vi "Main.vi"(11 "Module Admin":refnum<class "Delacor_lib_QMH_Module Admin.lvclass">) -> ()   [LabVIEW 2022 SP3, in "StateMachine.lvlib"]
doc: "This template is based off of the default DQMH. It implements the HSE Flavor of DQMH (see https://dokuwiki.hampel-soft.com/code/dqmh/hse-flavour) and adds a state machine to the module.\n\nThe state machine is based off of SSDC's (http://www.ssdc.co.uk/) state machine template. \n____\nHAMPEL SOFTWARE ENGINEERING v2.6.0 (2023-12-19 10:54)"
uses:
  StateMachine.lvlib
  <vilib>/Delacor/Delacor QMH/Libraries/Module Admin_class/Delacor_lib_QMH_Module Admin.lvclass
  HSE-SM/SM_States.ctl
  HSE-SM/SM_Transitions.ctl
  Module Data--cluster.ctl
  Libraries/hse-libraries/Source/hse-dqmh/Controls/Module Display Scenarios.ctl
  <vilib>/Delacor/Delacor QMH/Libraries/Module Admin_class/Delacor_lib_QMH_Module Admin.lvclass/Delacor_lib_QMH_Module Admin.ctl
  Configure Argument--cluster.ctl
  <vilib>/Delacor/Delacor QMH/Libraries/Message Queue_class/Delacor_lib_QMH_Message Queue.lvclass/Delacor_lib_QMH_Message Queue.ctl
  Prepare Argument--cluster.ctl
  Request UI Display Argument--cluster.ctl
  Request UI Display (Reply Payload)--cluster.ctl
  DEMO Inject Transition Argument--cluster.ctl
  Stop Argument--cluster.ctl
  <vilib>/Utility/miscctls.llb/LVPointTypeDef.ctl
  <vilib>/Delacor/Delacor QMH/Libraries/Message Queue_class/Delacor_lib_QMH_Enqueue Message (Single).vi
  <vilib>/Delacor/Delacor QMH/Libraries/Module Admin_class/Delacor_lib_QMH_Get External Launch.vi
  <vilib>/Utility/error.llb/Error Cluster From Error Code.vi
  <vilib>/ErrorRing/Error Ring.xnode
  <vilib>/Delacor/Delacor QMH/Libraries/Message Queue_class/Delacor_lib_QMH_Message Queue.lvclass
  Libraries/hse-libraries/Source/hse-configuration/config-ini/config-ini.lvclass
  <vilib>/Hampel Software Engineering/HSE Logger/hse-logger.lvlib
  Libraries/hse-libraries/Source/hse-dqmh/hse-dqmh.lvlib
  HSE-SM/HSE-State-Machine.lvlib
  Framework/UI Manager/UI Manager.lvlib
panel:
  in  "Nested Logic: Skip Polling?":bool caption="Skip Polling?"
  in  "Request Transition":T1
  in  "Polling Loop Signal":bool
  out "Current State":T2
  out "SM Exception":errorcluster
  out "error out":errorcluster
  # "The \"HSE State Machine Module\" serves as an example of how to use our HSE State Machine reference\narchitecture.\n\nThe module features a helper loop which hosts the state machine. Each state has a number of transitions\nit will process: Transitions can either lead to other states, be ignored, or even throw an error.\n\nBy default, states wait for transitions. Alternatively, there's the concept of \"polling states\".  Transitions \nare meant to be results of either the change of state of the system or triggered by user actions.\n\nUse the \"Request Transition\" enumerator to trigger transitions manually and observe how the state \nmachine reacts by watching the \"Current State\" indicator. Use the Skip Polling? and Polling Loop Signal \ncontrols accordingly to further manipulate the state machine."
  # "ENLARGE WINDOW TO SEE STATE CHART"
  # "See block diagram for details on this."
  # "Set this control to request a transition to the \nstate machine and observe its reaction with \nthe Current State indicator. \"Exit\" will close \nthe whole application."
  # "Set this control to \"true\" to satisfy the polling\ncondition and make the state machine leave\nthe polling state \"Polling for Signal Change\"."
  # "notice that the state machine doesn't allow the module to stop in every state and \nthat we didn't draw exception transitions."
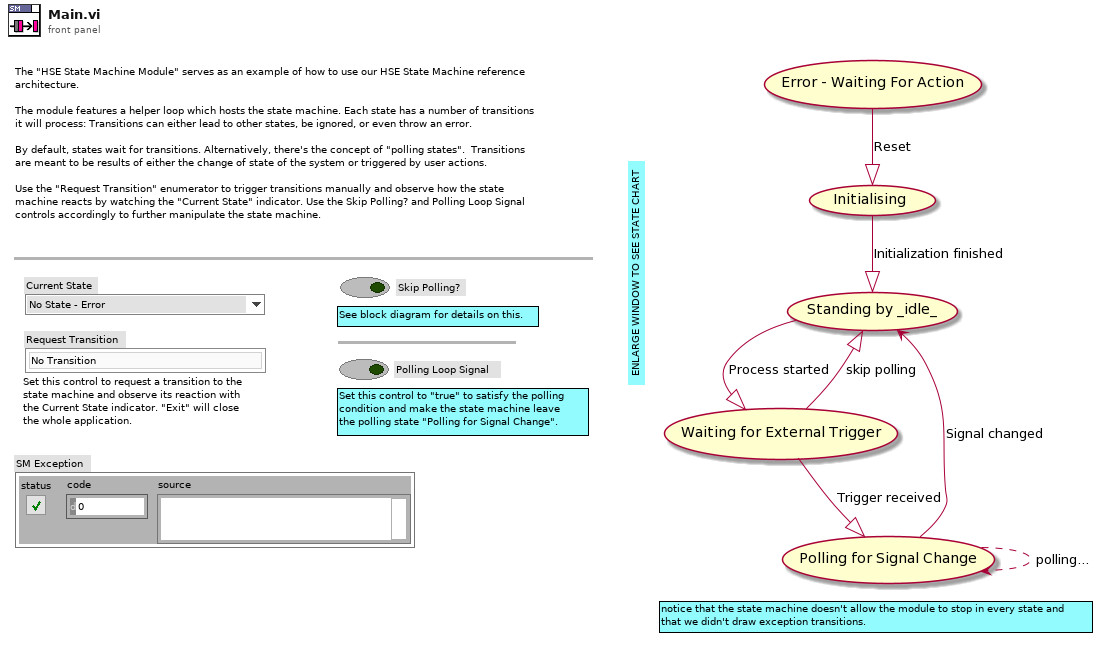
[diagram p1: front panel]
types:
  T1 = typedef "StateMachine.lvlib/HSE-State-Machine.lvlib/SM_Transitions.ctl" = enum16{"No Transition", "Exception", "Reset", "Initialization finished", "Process started", "Trigger detected", "Exit"}
  T2 = typedef "StateMachine.lvlib/HSE-State-Machine.lvlib/SM_States.ctl" = enum16{"No State - Error", "Error - Waiting For Action", "Initialising", "Standing by (idle)", "Waiting for External Trigger", "Polling for Signal Change", "Exiting"}
  T3 = typedef "StateMachine.lvlib/Request Events--cluster.ctl" = cluster{"Stop Module":refnum<user-event>, "Show Panel":refnum<user-event>, "Hide Panel":refnum<user-event>, "Get Module Execution Status":refnum<user-event>, "Show Diagram":refnum<user-event>, "Configure":refnum<user-event>, "Prepare":refnum<user-event>, "Request UI Display":refnum<user-event>, "DEMO Inject Transition":refnum<user-event>, "Exit EHL":refnum<user-event>}
  T4 = typedef "StateMachine.lvlib/Module Data--cluster.ctl" = cluster{"Scenario":T5}
  T5 = typedef "hse-dqmh.lvlib/Module Display Scenarios.ctl" = enum16{"Stand-Alone", "Managed"}
  T6 = typedef "StateMachine.lvlib/Stop Argument--cluster.ctl" = cluster{"Origin":string, "Exit via Stop Module Req?":bool, "Wait for Module to stop?":bool}
  T7 = enum32{"invalid lock state", "Not Locked", "Locked (No Password)", "Password-protected"}
  T8 = typedef "StateMachine.lvlib/Configure Argument--cluster.ctl" = cluster{"Boolean":bool}
  T9 = typedef "StateMachine.lvlib/Prepare Argument--cluster.ctl" = cluster{"Boolean":bool}
  T10 = typedef "StateMachine.lvlib/Request UI Display Argument--cluster.ctl" = cluster{"Scenario":T5, "Wait Notifier":refnum<notifier>, "wait for reply":bool}
  T11 = typedef "StateMachine.lvlib/DEMO Inject Transition Argument--cluster.ctl" = cluster{"Transition":T1, "Data":variant}
  T12 = typedef "LVPointTypeDef.ctl" = cluster{"Horizontal":i16, "Vertical":i16}
  T13 = enum32{"Invalid", "Standard", "Closed", "Hidden", "Minimized", "Maximized"}
  T14 = typedef "StateMachine.lvlib/Request UI Display (Reply Payload)--cluster.ctl" = cluster{"Accept?":bool, "error":errorcluster}
  T15 = typedef "StateMachine.lvlib/HSE-State-Machine.lvlib/SM Polling Actions--enum.ctl" = enum16{"Check transitions...", "Leave this state!"}
  T16 = typedef "hse-dqmh.lvlib/System Message Source.ctl" = enum16{"module", "application", "network"}
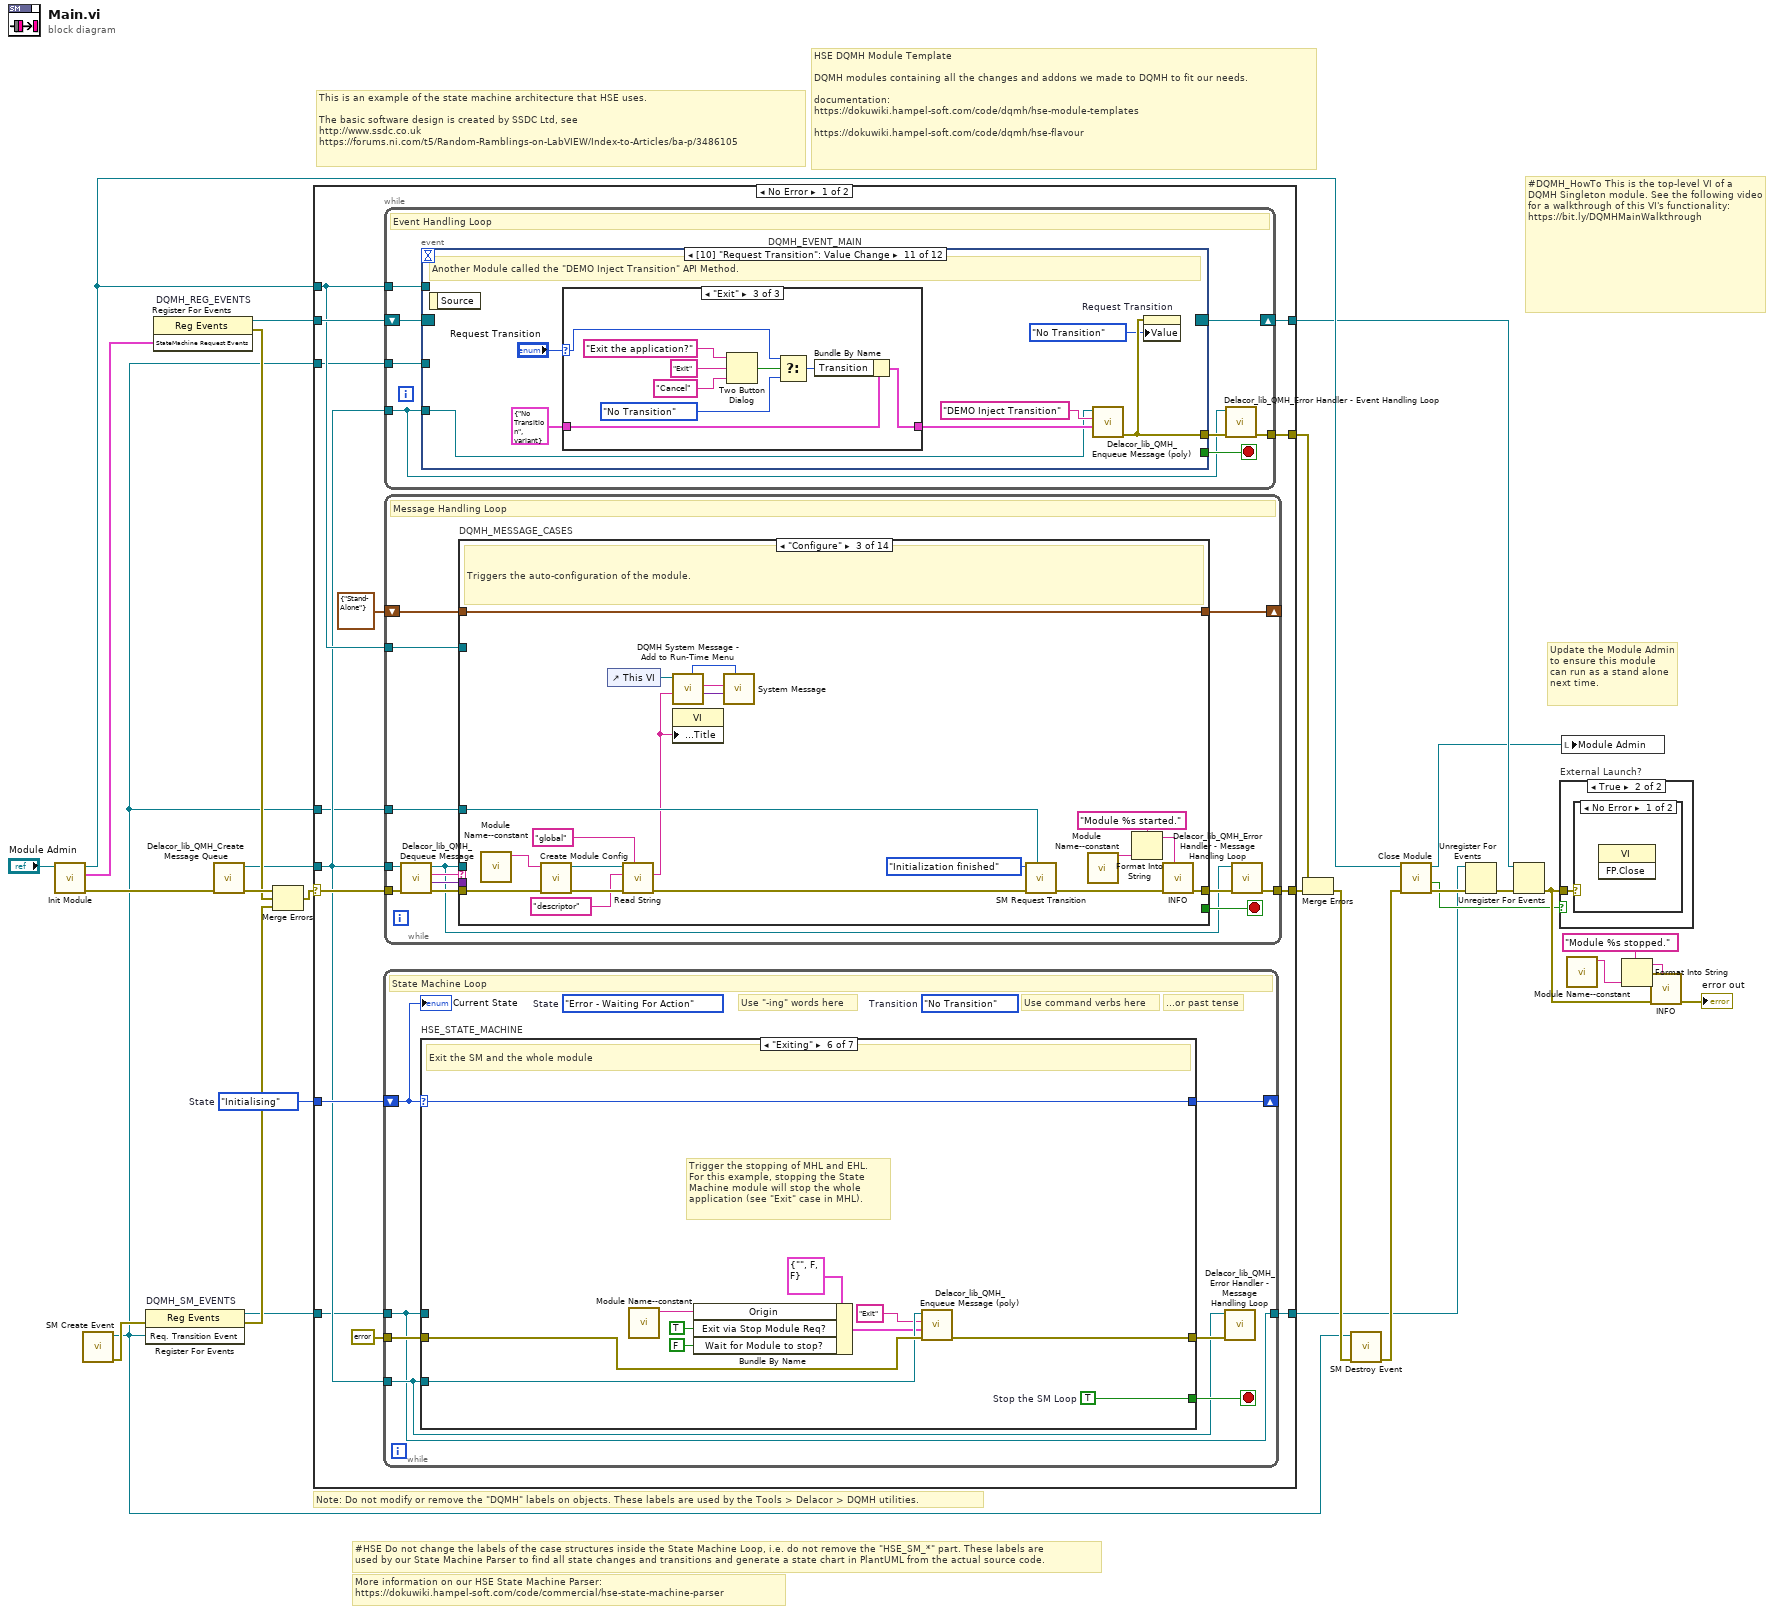
[diagram p0: block diagram]
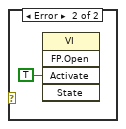
[diagram p3: hidden frame]
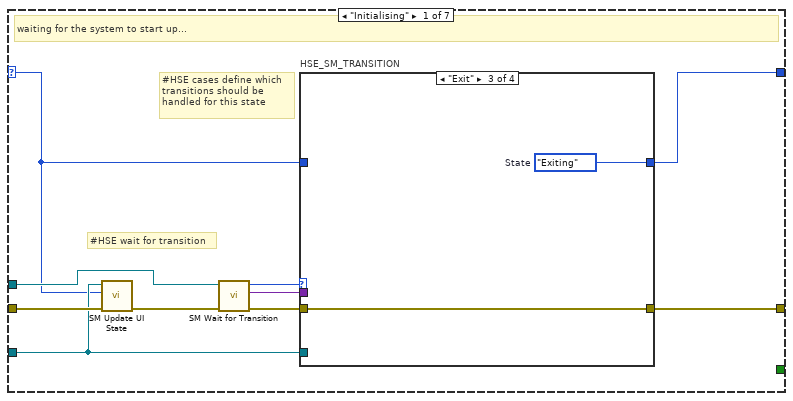
[diagram p4: hidden frame]
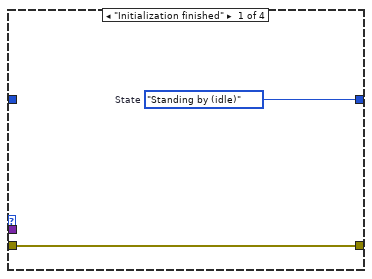
[diagram p5: hidden frame]
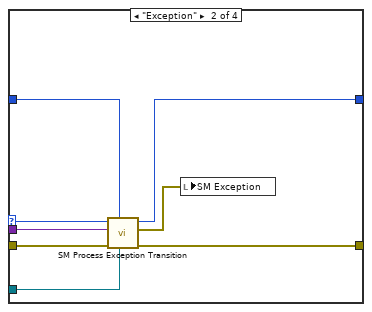
[diagram p6: hidden frame]
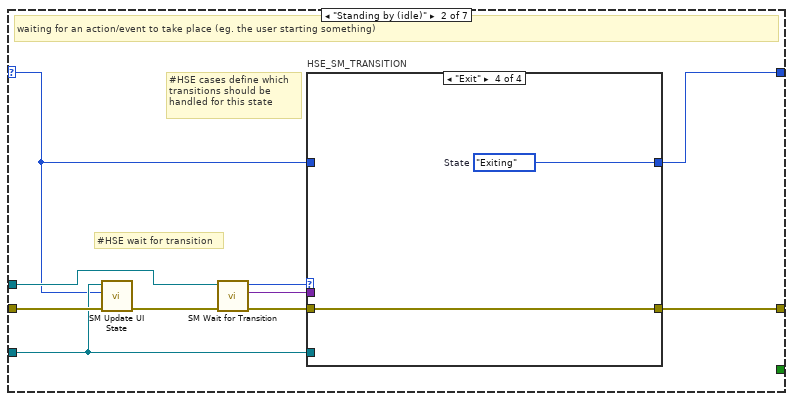
[diagram p8: hidden frame]
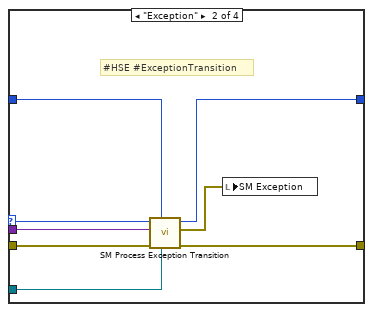
[diagram p10: hidden frame]
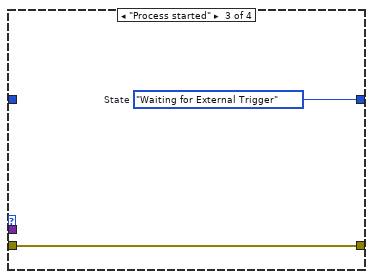
[diagram p11: hidden frame]
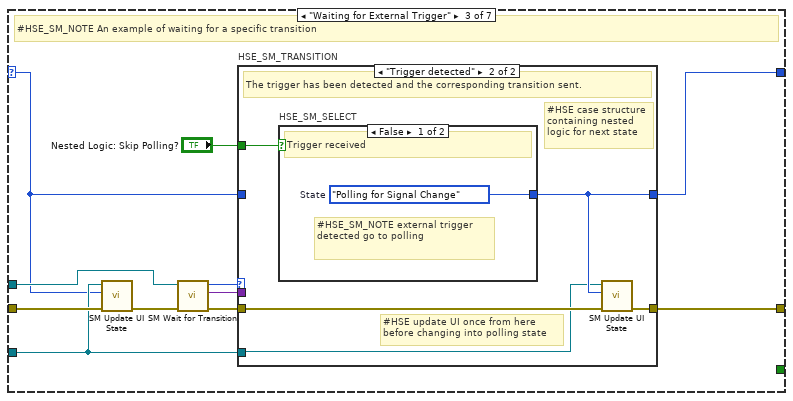
[diagram p12: hidden frame]
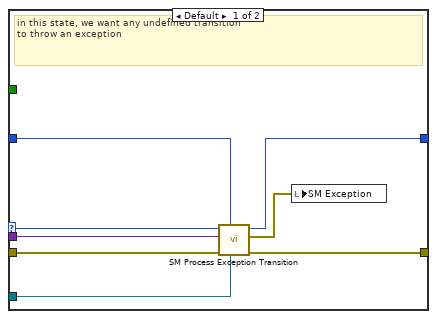
[diagram p13: hidden frame]
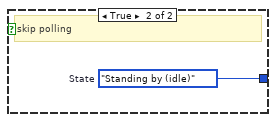
[diagram p14: hidden frame]
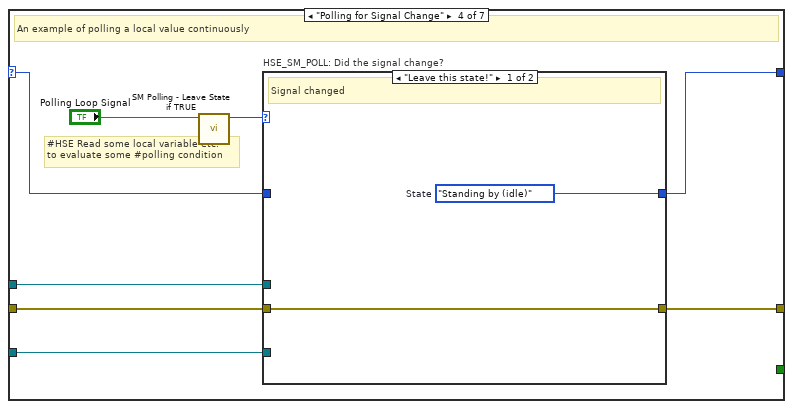
[diagram p15: hidden frame]
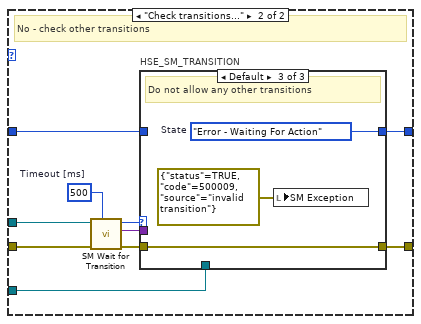
[diagram p16: hidden frame]
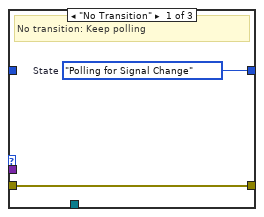
[diagram p17: hidden frame]
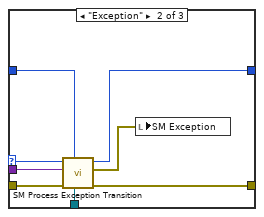
[diagram p18: hidden frame]
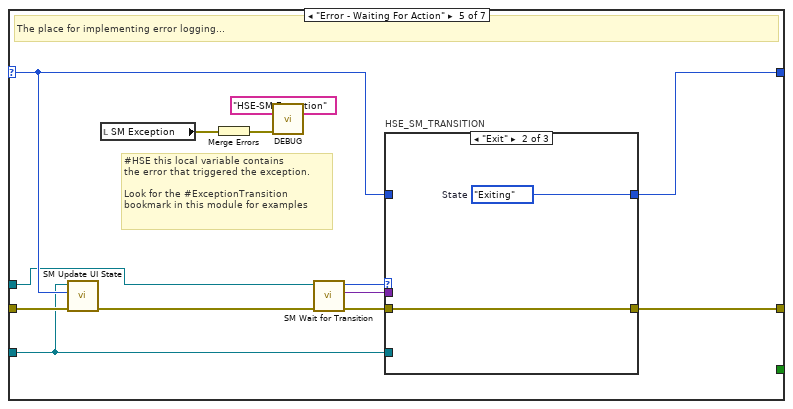
[diagram p19: hidden frame]
diagram:
  w12 = SM_States."Initialising"  # State
  # "More information on our HSE State Machine Parser: \nhttps://dokuwiki.hampel-soft.com/code/commercial/hse-state-machine-parser"
  # "#HSE Do not change the labels of the case structures inside the State Machine Loop, i.e. do not remove the \"HSE_SM_*\" part. These labels are\nused by our State Machine Parser to find all state changes and transitions and generate a state chart in PlantUML from the actual source code."
  # "HSE DQMH Module Template\n\nDQMH modules containing all the changes and addons we made to DQMH to fit our needs.\n\ndocumentation:\nhttps://dokuwiki.hampel-soft.com/code/dqmh/hse-module-templates\n\nhttps://dokuwiki.hampel-soft.com/code/dqmh/hse-flavour"
  # "This is an example of the state machine architecture that HSE uses. \n\nThe basic software design is created by SSDC Ltd, see \nhttp://www.ssdc.co.uk\nhttps://forums.ni.com/t5/Random-Ramblings-on-LabVIEW/Index-to-Articles/ba-p/3486105"
  # "#DQMH_HowTo This is the top-level VI of a DQMH Singleton module. See the following video for a walkthrough of this VI's functionality: https://bit.ly/DQMHMainWalkthrough"
  # "Note: Do not modify or remove the \"DQMH\" labels on objects. These labels are used by the Tools > Delacor > DQMH utilities."
  # "Update the Module Admin to ensure this module can run as a stand alone next time."
  n1 = call "Init Module.vi"("Singleton Module Admin in"="Module Admin") -> ("error out"=w27:errorcluster, "StateMachine Request Events"=w11:T3, "Singleton Module Admin out"=w23:refnum<class "Delacor_lib_QMH_Module Admin.lvclass">)  [unwired: 8 in]
  n2 = call "SM Create Event.vi"() -> ("error out"=w8:errorcluster, "Req. Transition Event"=w5:refnum<user-event>)  [unwired: 10 in]
  n3 = register-events "DQMH_SM_EVENTS"(error in=w8, w5) -> (reference out=w10:refnum<event-registration>, error out=w29:errorcluster)  [unwired: 1 in]
  n4 = register-events "DQMH_REG_EVENTS"(w11) -> (reference out=w21:refnum<event-registration>, error out=w24:errorcluster)  [unwired: 2 in]
  n5 = call <vilib>:"Delacor_lib_QMH_Create Message Queue.vi"("error in"=w27) -> ("error out"=w25:errorcluster, "Message Queue"=w20:refnum<class "Delacor_lib_QMH_Message Queue.lvclass">)  [unwired: 9 in]
  n6 = Merge Errors(w25, w24, w29) -> (w9:errorcluster)
  n7 = case shown="No Error" w9 {
    selector: w9 -> [w41 w468]
    tunnel: [w43 w467] -> w28
    tunnel: [w40 w473] -> w22
    tunnel: w21 -> [w38 w473]
    tunnel: w20 -> [w35 w466]
    tunnel: [w42 _] -> w26
    tunnel: w23 -> [w37 w469]
    tunnel: w12 -> [w36 _]
    tunnel: w10 -> [w34 w465]
    tunnel: w5 -> [w32 _]
    tunnel: w5 -> [w31 _]
    tunnel: [w30 w465] -> w1
    frame No Error {
      n8 = while {
        shift-right: [w49] -> _
        shift-left: w36 -> [w50]
        tunnel: w35 -> [w45]
        tunnel: w34 -> [w44]
        tunnel: errorcluster {"status"=FALSE, "code"=0, "source"=""} ("error out") -> [w46]
        tunnel: [w44] -> w30
        stop <- w48 stop-if-true
        (unwired) SM_States."Error - Waiting For Action"  # State
        (unwired) SM_Transitions."No Transition"  # Transition
        # "...or past tense"
        # "Use command verbs here"
        # "Use \"-ing\" words here"
        # "State Machine Loop"
        n9 = case "HSE_STATE_MACHINE" shown="\"Exiting\"" w50 {
          selector: w50 -> [w51 w75 w99 w125 w161 w184 _]
          tunnel: [w56 w80 w105 w131 w162 w184 w189] -> w49
          tunnel: [_ _ _ _ _ w187 w191] -> w48
          tunnel: w45 -> [w52 w76 w101 w129 w158 w186 _]
          tunnel: [w55 w79 w104 w130 w164 w185 errorcluster {"status"=TRUE, "code"=500001, "source"="SM called \"No State\"!"} ("error out")] -> w47
          tunnel: w44 -> [w53 w77 w102 w128 w160 _ _]
          tunnel: w46 -> [w60 w84 w109 w132 w170 w188 _]
          frame "Initialising" {
            # "#HSE cases define which\ntransitions should be \nhandled for this state"
            # "#HSE wait for transition"
            # "waiting for the system to start up..."
            n10 = call "SM Update UI State.vi"("error in (no error)"=w60, "State"=w51, "Message Queue In"=w52) -> ("error out"=w54:errorcluster)  [unwired: 7 in, 1 out]
            n11 = call "SM Wait for Transition.vi"("error in (no error)"=w54, "Event Registration Refnum"=w53) -> ("error out"=w58:errorcluster, "Data"=w57:variant, "Transition"=w59:T1)  [unwired: 7 in]
            n12 = case "HSE_SM_TRANSITION" shown="\"Exit\"" w59 {
              selector: w59 -> [_ w64 _ _]
              tunnel: w58 -> [w62 w70 w72 w73]
              tunnel: w57 -> [_ w69 _ _]
              tunnel: [w61 w68 w71 w74] -> w56
              tunnel: [w62 w67 w72 w73] -> w55
              tunnel: w52 -> [_ w65 _ _]
              tunnel: w51 -> [_ w63 _ w74]
              frame "Initialization finished" {
                w61 = SM_States."Standing by (idle)"  # State
              }
              frame "Exception" {
                n13 = call "SM Process Exception Transition.vi"("Message Queue In"=w65, "Exception State"=w63, "error in (no error)"=w70, "Data"=w69, "Exception Transition"=w64) -> ("error out"=w67:errorcluster, "Exception"=w66:errorcluster, "State"=w68:T2)  [unwired: 4 in]
                n14 = local write "SM Exception"(w66) -> ()
              }
              frame "Exit" {
                w71 = SM_States."Exiting"  # State
              }
              frame Default {
                # "we intentionally want to ignore silently every other transition\nin this case"
              }
            }
          }
          frame "Standing by (idle)" {
            # "#HSE cases define which\ntransitions should be \nhandled for this state"
            # "#HSE wait for transition"
            # "waiting for an action/event to take place (eg. the user starting something)"
            n15 = call "SM Update UI State.vi"("error in (no error)"=w84, "State"=w75, "Message Queue In"=w76) -> ("error out"=w78:errorcluster)  [unwired: 7 in, 1 out]
            n16 = call "SM Wait for Transition.vi"("error in (no error)"=w78, "Event Registration Refnum"=w77) -> ("error out"=w82:errorcluster, "Data"=w81:variant, "Transition"=w83:T1)  [unwired: 7 in]
            n17 = case "HSE_SM_TRANSITION" shown="\"Exit\"" w83 {
              selector: w83 -> [_ w88 _ _]
              tunnel: w82 -> [w85 w94 w96 w97]
              tunnel: w81 -> [_ w93 _ _]
              tunnel: [w86 w92 w95 w98] -> w80
              tunnel: [w85 w91 w96 w97] -> w79
              tunnel: w76 -> [_ w89 _ _]
              tunnel: w75 -> [w86 w87 _ _]
              frame Default {
                # "we intentionally want to ignore silently every other transition\nin this case"
              }
              frame "Exception" {
                # "#HSE #ExceptionTransition"
                n18 = call "SM Process Exception Transition.vi"("Message Queue In"=w89, "Exception State"=w87, "error in (no error)"=w94, "Data"=w93, "Exception Transition"=w88) -> ("error out"=w91:errorcluster, "Exception"=w90:errorcluster, "State"=w92:T2)  [unwired: 4 in]
                n19 = local write "SM Exception"(w90) -> ()
              }
              frame "Process started" {
                w95 = SM_States."Waiting for External Trigger"  # State
              }
              frame "Exit" {
                w98 = SM_States."Exiting"  # State
              }
            }
          }
          frame "Waiting for External Trigger" {
            # "#HSE_SM_NOTE An example of waiting for a specific transition"
            n20 = call "SM Update UI State.vi"("error in (no error)"=w109, "State"=w99, "Message Queue In"=w101) -> ("error out"=w103:errorcluster)  [unwired: 7 in, 1 out]
            n21 = call "SM Wait for Transition.vi"("error in (no error)"=w103, "Event Registration Refnum"=w102) -> ("error out"=w107:errorcluster, "Data"=w106:variant, "Transition"=w108:T1)  [unwired: 7 in]
            n22 = case "HSE_SM_TRANSITION" shown="\"Trigger detected\"" w108 {
              selector: w108 -> [w112 _]
              tunnel: w107 -> [w117 w122]
              tunnel: w106 -> [w116 _]
              tunnel: [w111 w120] -> w105
              tunnel: [w115 w121] -> w104
              tunnel: w101 -> [w113 w119]
              tunnel: "Nested Logic: Skip Polling?" -> [_ w118]
              tunnel: w99 -> [w110 _]
              frame Default {
                # "in this state, we want any undefined transition \nto throw an exception"
                n23 = call "SM Process Exception Transition.vi"("Message Queue In"=w113, "Exception State"=w110, "error in (no error)"=w117, "Data"=w116, "Exception Transition"=w112) -> ("error out"=w115:errorcluster, "Exception"=w114:errorcluster, "State"=w111:T2)  [unwired: 4 in]
                n24 = local write "SM Exception"(w114) -> ()
              }
              frame "Trigger detected" {
                # "#HSE case structure\ncontaining nested \nlogic for next state"
                # "#HSE update UI once from here\nbefore changing into polling state"
                # "The trigger has been detected and the corresponding transition sent."
                n25 = case "HSE_SM_SELECT" shown="False" w118 {
                  tunnel: [w123 w124] -> w120
                  frame False {
                    w123 = SM_States."Polling for Signal Change"  # State
                    # "#HSE_SM_NOTE external trigger detected go to polling"
                    # "Trigger received"
                  }
                  frame True {
                    w124 = SM_States."Standing by (idle)"  # State
                    # "skip polling"
                  }
                }
                n26 = call "SM Update UI State.vi"("error in (no error)"=w122, "State"=w120, "Message Queue In"=w119) -> ("error out"=w121:errorcluster)  [unwired: 7 in, 1 out]
              }
            }
          }
          frame "Polling for Signal Change" {
            # "#HSE Read some local variable etc. \nto evaluate some #polling condition"
            # "An example of polling a local value continuously"
            n27 = call "SM Polling - Leave State if TRUE.vi"("Boolean Condition"="Polling Loop Signal") -> ("Polling Action"=w127:T15)  [unwired: 10 in]
            n28 = case "HSE_SM_POLL: Did the signal change?" shown="\"Leave this state!\"" w127 {
              tunnel: w132 -> [w134 w144]
              tunnel: [w133 w140] -> w131
              tunnel: [w134 w139] -> w130
              tunnel: w129 -> [_ w138]
              tunnel: w128 -> [_ w137]
              tunnel: w125 -> [_ w135]
              frame "Leave this state!" {
                w133 = SM_States."Standing by (idle)"  # State
                # "Signal changed"
              }
              frame "Check transitions..." {
                w136 = 500  # Timeout [ms]
                # "No - check other transitions"
                n29 = call "SM Wait for Transition.vi"("Timeout [ms]"=w136, "error in (no error)"=w144, "Event Registration Refnum"=w137) -> ("error out"=w142:errorcluster, "Data"=w141:variant, "Transition"=w143:T1)  [unwired: 6 in]
                n30 = case "HSE_SM_TRANSITION" shown="Default" w143 {
                  selector: w143 -> [_ w149 _]
                  tunnel: w142 -> [w145 w154 w156]
                  tunnel: w141 -> [_ w153 _]
                  tunnel: [w146 w148 w155] -> w140
                  tunnel: [w145 w152 w156] -> w139
                  tunnel: w138 -> [_ w150 _]
                  tunnel: w135 -> [_ w147 _]
                  frame "No Transition" {
                    w146 = SM_States."Polling for Signal Change"  # State
                    # "No transition: Keep polling"
                  }
                  frame "Exception" {
                    n31 = call "SM Process Exception Transition.vi"("Message Queue In"=w150, "Exception State"=w147, "error in (no error)"=w154, "Data"=w153, "Exception Transition"=w149) -> ("error out"=w152:errorcluster, "Exception"=w151:errorcluster, "State"=w148:T2)  [unwired: 4 in]
                    n32 = local write "SM Exception"(w151) -> ()
                  }
                  frame Default {
                    w155 = SM_States."Error - Waiting For Action"  # State
                    # "Do not allow any other transitions"
                    n33 = local write "SM Exception"(errorcluster {"status"=TRUE, "code"=500009, "source"="invalid transition"} ("SM Exception")) -> ()
                  }
                }
              }
            }
          }
          frame "Error - Waiting For Action" {
            # "#HSE this local variable contains\nthe error that triggered the exception.\n\nLook for the #ExceptionTransition \nbookmark in this module for examples"
            # "The place for implementing error logging..."
            n34 = call "SM Update UI State.vi"("error in (no error)"=w170, "State"=w161, "Message Queue In"=w158) -> ("error out"=w166:errorcluster)  [unwired: 7 in, 1 out]
            n35 = local read "SM Exception"() -> (w169:errorcluster)
            n36 = Merge Errors(w169) -> (w168:errorcluster)
            n37 = call <vilib>:"DEBUG.vi"("Message"="HSE-SM Exception", "error in"=w168) -> ()  [unwired: 9 in, 1 out]
            n38 = call "SM Wait for Transition.vi"("error in (no error)"=w166, "Event Registration Refnum"=w160) -> ("error out"=w163:errorcluster, "Data"=w159:variant, "Transition"=w165:T1)  [unwired: 7 in]
            n39 = case "HSE_SM_TRANSITION" shown="\"Exit\"" w165 {
              tunnel: [w171 w173 w176] -> w164
              tunnel: w163 -> [w171 w173 w176]
              tunnel: [w172 w174 w177] -> w162
              tunnel: w161 -> [w172 _ _]
              tunnel: w159 -> [_ _ _]
              tunnel: w158 -> [_ _ _]
              frame Default {
                # "just silently ignore any other transitions"
              }
              frame "Exit" {
                w174 = SM_States."Exiting"  # State
              }
              frame "Reset" {
                w177 = SM_States."Initialising"  # State
                "SM Exception" <- errorcluster {"status"=FALSE, "code"=0, "source"=""} ("SM Exception")
              }
            }
          }
          frame "Exiting" {
            w187 = TRUE  # Stop the SM Loop
            # "Trigger the stopping of MHL and EHL.\nFor this example, stopping the State\nMachine module will stop the whole\napplication (see \"Exit\" case in MHL)."
            # "Exit the SM and the whole module"
            n40 = call "Module Name--constant.vi"() -> ("Module Name"=w178:string)  [unwired: 11 in]
            n41 = Bundle By Name(cluster=T6 {"Origin"="", "Exit via Stop Module Req?"=FALSE, "Wait for Module to stop?"=FALSE} ("Stop Argument"), "Origin"=w178, "Exit via Stop Module Req?"=TRUE, "Wait for Module to stop?"=FALSE) -> (w181:T6)
            n42 = call-poly <vilib>:"Delacor_lib_QMH_Enqueue Message (poly).vi"("error in"=w188, "Message Data"=w181, "Message"="Exit", "Message Queue in"=w186) -> ("error out"=w185:errorcluster)  [unwired: 6 in, 1 out]
          }
          frame "No State - Error" {
            w189 = SM_States."Error - Waiting For Action"  # State
            w191 = FALSE  # Exit
          }
        }
        n43 = call-dynamic "Delacor_lib_QMH_Error Handler - Message Handling Loop.vi"("error in"=w47, "Message Queue in"=w45) -> ()  [unwired: 8 in, 2 out]
        "Current State" <- w50
      }
      n44 = while {
        tunnel: w35 -> [w193]
        shift-right: [w196] -> w40
        shift-left: w38 -> [w197]
        tunnel: [w198] -> w42
        tunnel: w37 -> [w194]
        tunnel: w31 -> [w192]
        stop <- w195 stop-if-true
        # "Event Handling Loop"
        n45 = event "DQMH_EVENT_MAIN" shown="[10] \"Request Transition\": Value Change" {
          selector: w197 -> [_ _ _ _ _ _ _ _ _ _ _ _]
          dyn-events: [_ _ _ _ _ _ _ _ _ _ _ _] -> w196
          timeout: _ -> [_ _ _ _ _ _ _ _ _ _ _ _]
          tunnel: [_ _ _ _ _ _ _ _ _ _ _ w280] -> w195
          tunnel: w193 -> [_ _ _ _ _ w221 w235 w241 w249 w256 w258 _]
          tunnel: [_ _ w205 _ w217 w223 w231 w237 w245 w252 w260 _] -> w199
          tunnel: w194 -> [_ _ _ _ _ w220 _ _ _ _ _ _]
          tunnel: w192 -> [_ _ _ _ w215 w218 _ _ _ _ _ _]
          event User Event {
            # "Show the panel of this VI, and send a status updated message to let listeners know."
            # "Another Module called the \"Show Panel\" API Method."
            n46 = event-data() -> ()  [unwired: 1 in, 1 out]
            n47 = control-ref of="This VI"() -> (w201:refnum<vi>)
            n48 = call "Open VI Panel.vi"("VI"=w201) -> ()  [unwired: 10 in, 1 out]
            n49 = call "Status Updated.vi"("Status"="Panel shown." ("format string")) -> ()  [unwired: 10 in, 1 out]
          }
          event User Event {
            # "Hide the panel of this VI, and send a status updated message to let listeners know."
            # "Another Module called the \"Hide Panel\" API Method."
            n50 = event-data() -> ()  [unwired: 1 in, 1 out]
            n51 = control-ref of="This VI"() -> (w203:refnum<vi>)
            n52 = call "Hide VI Panel.vi"("VI"=w203) -> ()  [unwired: 10 in, 1 out]
            n53 = call "Status Updated.vi"("Status"="Panel hidden." ("format string")) -> ()  [unwired: 10 in, 1 out]
          }
          event User Event {
            # "Another Module called the \"Get Module Execution Status\" API Method."
            n54 = event-data() -> ()  [unwired: 1 in, 1 out]
            n55 = call "Update Module Execution Status.vi"("Running?"=TRUE) -> ("error out"=w205:errorcluster)  [unwired: 10 in]
          }
          event User Event {
            # "Another Module called the \"Show Diagram\" API Method. This event is used for debugging."
            n56 = event-data() -> ()  [unwired: 1 in, 1 out]
            n57 = disable-structure shown="RUN_TIME_ENGINE==False" {
              frame condition #0 (active) {
                # "functionality not available in exe"
                n58 = invoke class="VI" method="Lock State.Get"() -> (error out=w211:errorcluster, "Get Lock State"=w210:T7, "pwd in cache"=w207:bool)  [unwired: 4 in, 1 out]
                n59 = Equal?(x=T7."Password-protected", y=w210) -> (x = y?=w208:bool)
                n60 = Compound Arithmetic op=AND(w208, invert w207) -> (w206:bool)
                n61 = case shown="False" w206 {
                  tunnel: w211 -> [w214 _]
                  frame False {
                    n62 = property class="VI"(error in=w214, "BDWin.Open"=TRUE ("Block Diagram Window:Open")) -> ()  [unwired: 1 in, 2 out]
                    n63 = call "Status Updated.vi"("Status"="Block Diagram shown." ("format string")) -> ()  [unwired: 10 in, 1 out]
                  }
                  frame True {
                    # "Password-protected VI, and the password is not in the cache. Do not show the diagram."
                  }
                }
              }
              frame condition #1 {
              }
            }
          }
          event User Event {
            # "Don't use normal DQMH stop procedure, but trigger the \"Exit\" transition.\nThe state machine will decide if the module should actually stop. The SM\nwill then trigger stopping the MHL which triggers stopping the EHL in turn\n(see the \"Exit EHL\" event case)."
            # "Another Module called the \"Stop Module\" API Method  or the Message Handling Loop below."
            n64 = event-data() -> ()  [unwired: 1 in, 3 out]
            n65 = call "SM Request Transition.vi"("Req. Transition"=w215, "Transition"=SM_Transitions."Exit") -> ("error out"=w217:errorcluster)  [unwired: 9 in]
          }
          event Panel Close? {
            w222 = TRUE  # Discard the event, the MHL is responsible for closing and stopping this VI.
            # "don't use normal DQMH stop procedure, but request the Exit transition the state machine will decide, if the module should actually stop"
            # "Hide the panel or send the 'Exit' message if the user clicks the 'X' on the module main VI panel."
            n66 = event-data() -> ()  [unwired: 1 in, 1 out]
            n67 = property class="Module Admin"(reference=w220) -> ("Accessors:External Launch"=w219:bool)  [unwired: 1 in, 2 out]
            n68 = case shown="False" w219 {
              tunnel: w221 -> [_ _]
              tunnel: [_ w229] -> w223
              tunnel: w218 -> [_ w227]
              frame True {
                w225 = "Panel hidden."  # Status
                # "If externally launched, clicking the 'X' hides the panel, but doesn't close it."
                n69 = control-ref of="This VI"() -> (w226:refnum<vi>)
                n70 = call "Hide VI Panel.vi"("VI"=w226) -> ("error out"=w224:errorcluster)  [unwired: 10 in]
                n71 = call "Status Updated.vi"("error in (no error)"=w224, "Status"=w225) -> ()  [unwired: 9 in, 1 out]
              }
              frame False {
                # "If run as a stand-alone VI, clicking the panel 'X' requests the State Machine to Exit."
                n72 = call "SM Request Transition.vi"("Req. Transition"=w227, "Transition"=SM_Transitions."Exit") -> ("error out"=w229:errorcluster)  [unwired: 9 in]
              }
            }
            n73 = event-data("Discard?"=w222) -> ()  [unwired: 1 in, 1 out]
          }
          event User Event {
            # "Another Module called the \"Configure\" API Method."
            n74 = event-data() -> ("Boolean"=w230:bool)  [unwired: 1 in]
            n75 = Bundle(cluster=T8 {"Boolean"=FALSE} ("Configure Argument"), "Boolean"=w230) -> (w232:T8)
            n76 = call-poly <vilib>:"Delacor_lib_QMH_Enqueue Message (poly).vi"("Message Data"=w232, "Message"="Configure", "Message Queue in"=w235) -> ("error out"=w231:errorcluster)  [unwired: 7 in, 1 out]
          }
          event User Event {
            # "Another Module called the \"Prepare\" API Method."
            n77 = event-data() -> ("Boolean"=w236:bool)  [unwired: 1 in]
            n78 = Bundle(cluster=T9 {"Boolean"=FALSE} ("Prepare Argument"), "Boolean"=w236) -> (w238:T9)
            n79 = call-poly <vilib>:"Delacor_lib_QMH_Enqueue Message (poly).vi"("Message Data"=w238, "Message"="Prepare", "Message Queue in"=w241) -> ("error out"=w237:errorcluster)  [unwired: 7 in, 1 out]
          }
          event User Event {
            # "Another Module called the \"Request UI Display\" API Method."
            n80 = event-data() -> ("Scenario"=w244:T5, "Wait Notifier"=w243:refnum<notifier>, "wait for reply"=w242:bool)  [unwired: 1 in]
            n81 = Bundle(cluster=T10 {"Scenario"=enum."Stand-Alone", "Wait Notifier"=refnum, "wait for reply"=FALSE} ("Request UI Display Argument"), "Scenario"=w244, "Wait Notifier"=w243, "wait for reply"=w242) -> (w246:T10)
            n82 = call-poly <vilib>:"Delacor_lib_QMH_Enqueue Message (poly).vi"("Message Data"=w246, "Message"="Request UI Display", "Message Queue in"=w249) -> ("error out"=w245:errorcluster)  [unwired: 7 in, 1 out]
          }
          event User Event {
            # "Another Module called the \"DEMO Inject Transition\" API Method."
            n83 = event-data() -> ("Transition"=w251:T1, "Data"=w250:variant)  [unwired: 1 in]
            n84 = Bundle(cluster=T11 {"Transition"=enum."No Transition", "Data"=variant} ("DEMO Inject Transition Argument"), "Transition"=w251, "Data"=w250) -> (w253:T11)
            n85 = call-poly <vilib>:"Delacor_lib_QMH_Enqueue Message (poly).vi"("Message Data"=w253, "Message"="DEMO Inject Transition", "Message Queue in"=w256) -> ("error out"=w252:errorcluster)  [unwired: 7 in, 1 out]
          }
          event Value Change {
            # "Another Module called the \"DEMO Inject Transition\" API Method."
            n86 = event-data() -> ()  [unwired: 1 in, 1 out]
            n87 = case shown="\"Exit\"" "Request Transition" {
              selector: "Request Transition" -> [w266 w267 w271]
              tunnel: [w264 w269 w275] -> w262
              tunnel: T11 {"Transition"=enum."No Transition", "Data"=variant} ("DEMO Inject Transition Argument") -> [w265 w270 w276]
              frame Default {
                n88 = Bundle By Name(cluster=w265, "Transition"=w266) -> (w264:T11)
              }
              frame "Exception" {
                n89 = Bundle By Name(cluster=w270, "Transition"=w267, "Data"=errorcluster {"status"=TRUE, "code"=500002, "source"="Exception State"} ("error out")) -> (w269:T11)
              }
              frame "Exit" {
                n90 = Two Button Dialog(message="Exit the application?", 1:"Cancel" ("F button name (\"Cancel\")"), 2:"Exit" ("T button name (\"OK\")")) -> (T button?=w274:bool)
                n91 = Select(t=w271, s=w274, f=SM_Transitions."No Transition" ("Request Transition")) -> (s? t:f=w273:T1)
                n92 = Bundle By Name(cluster=w276, "Transition"=w273) -> (w275:T11)
              }
            }
            n93 = call-poly <vilib>:"Delacor_lib_QMH_Enqueue Message (poly).vi"("Message Data"=w262, "Message"="DEMO Inject Transition", "Message Queue in"=w258) -> ("error out"=w260:errorcluster)  [unwired: 7 in, 1 out]
            n94 = property on="Request Transition" class="Enum (strict)"(error in=w260, "Value"=SM_Transitions."No Transition" ("Request Transition")) -> ()  [unwired: 1 in, 2 out]
          }
          event User Event {
            w280 = TRUE  # Stop the EHL Loop
            # "This MHL called the \"Exit EHL\" private API Method."
            n95 = event-data() -> ()  [unwired: 1 in, 1 out]
          }
        }
        n96 = call-dynamic "Delacor_lib_QMH_Error Handler - Event Handling Loop.vi"("error in"=w199, "Message Queue in"=w193) -> ("dup error in"=w198:errorcluster)  [unwired: 8 in, 1 out]
      }
      n97 = while {
        tunnel: w35 -> [w284]
        shift-right: [w288] -> _
        shift-left: T4 {"Scenario"=enum."Stand-Alone"} ("Data Cluster") -> [w289]
        tunnel: w41 -> [w292]
        tunnel: [w290] -> w43
        tunnel: w37 -> [w282]
        tunnel: w32 -> [w281]
        stop <- w287 stop-if-true
        # "Message Handling Loop"
        n98 = call-dynamic "Delacor_lib_QMH_Dequeue Message.vi"("error in"=w292, "Message Queue in"=w284) -> ("error out"=w291:errorcluster, "Message Data"=w285:variant, "Message"=w286:string, "Message Queue out"=w283:refnum<class "Delacor_lib_QMH_Message Queue.lvclass">)  [unwired: 6 in]
        n99 = case "DQMH_MESSAGE_CASES" shown="\"Configure\"" w286 {
          selector: w286 -> [_ _ _ _ _ _ _ _ _ _ _ _ _ w452]
          tunnel: w283 -> [_ _ _ _ w353 _ _ _ _ _ _ w420 w442 _]
          tunnel: w291 -> [w312 w316 w323 w339 w366 w372 w379 w390 w400 w408 w414 w427 w450 w454]
          tunnel: [w297 w316 w335 w340 w359 w372 w374 w389 w394 w411 w414 w423 w449 w455] -> w293
          tunnel: w289 -> [w301 w315 w336 w343 w365 w371 w378 w388 w399 w412 w413 w422 w448 w453]
          tunnel: [w301 w315 w336 w343 w358 w371 w378 w388 w399 w412 w413 w422 w448 w453] -> w288
          tunnel: [_ _ _ _ _ _ _ _ _ _ _ _ w447 _] -> w287
          tunnel: w285 -> [_ _ _ _ w364 _ w376 _ w398 _ _ w421 w446 _]
          tunnel: w282 -> [w302 _ _ _ _ _ _ _ _ _ _ w419 w443 _]
          tunnel: w281 -> [_ _ w329 _ _ _ _ _ w391 w409 _ _ _ _]
          frame "Initialize" {
            # "Initialize - Any operation that needs to be done before the module can receive messages. Synchronize Caller Events.vi will inform Start Module.vi that the module has launched and is ready to receive messages. Module Did Init.vi will broadcast that the module initialized."
            n100 = call "Synchronize Caller Events.vi"("error in (no error)"=w312, "Singleton Module Admin in"=w302) -> ("error out"=w311:errorcluster, "Singleton Module Admin out"=w299:refnum<class "Delacor_lib_QMH_Module Admin.lvclass">)  [unwired: 8 in]
            n101 = property class="Module Admin"(reference=w299) -> ("Accessors:External Launch"=w306:bool)  [unwired: 1 in, 2 out]
            n102 = property on="Pane" class="Pane"("Origin"=T12 {"Horizontal"=0, "Vertical"=0}) -> ()  [unwired: 2 in, 2 out]
            n103 = call "Module Name--constant.vi"() -> ("Module Name"=w294:string)  [unwired: 11 in]
            n104 = call "Module Did Init.vi"("error in (no error)"=w311, "Initialized?"=TRUE, "Origin"=w294) -> ("error out"=w310:errorcluster)  [unwired: 8 in]
            n105 = Select(t=T13."Hidden" ("State"), s=w306, f=T13."Standard" ("State")) -> (s? t:f=w303:T13)
            n106 = call "Module Name--constant.vi"() -> ("Module Name"=w309:string)  [unwired: 11 in]
            n107 = property class="VI"("Front Panel.Title"=w309) -> (reference out=w308:refnum<vi>, error out=w314:errorcluster)  [unwired: 2 in]
            n108 = invoke class="VI" method="FP.Open"(reference=w308, error in=w314, "State"=w303) -> (reference out=w307:refnum<vi>, error out=w313:errorcluster)  [unwired: 2 in, 3 out]
            n109 = Format Into String(format string="Module %s started.", w294) -> (resulting string=w295:string)  [unwired: 2 in, 1 out]
            n110 = call <vilib>:"INFO.vi"("Message"=w295, "error in"=w310) -> ("error out"=w297:errorcluster)  [unwired: 9 in]
            n111 = invoke class="VI" method="FP.Center"(reference=w307, error in=w313) -> ()  [unwired: 1 in, 3 out]
          }
          frame "---HSE---" {
            # "Separator -- The following cases handle messages specific to the HSE DQMH Flavour"
          }
          frame "Configure" {
            # "Triggers the auto-configuration of the module."
            n112 = call "Module Name--constant.vi"() -> ("Module Name"=w320:string)  [unwired: 11 in]
            n113 = call "Create Module Config.vi"("error in"=w323, "DQMH Module Name"=w320) -> ("error out"=w322:errorcluster, "config-ini out"=w321:refnum<class "config-ini.lvclass">)  [unwired: 8 in]
            n114 = control-ref of="This VI"() -> (w324:refnum<vi>)
            n115 = call-dynamic "Read String.vi"("Section"="global", "error in"=w322, "Key"="descriptor", "config-base in"=w321) -> ("error out"=w331:errorcluster, "Value"=w317:string)  [unwired: 5 in, 1 out]
            n116 = call "DQMH System Message - Add to Run-Time Menu.vi"("Module Descriptor"=w317, "Main VI Reference"=w324) -> ("Payload"=w326:variant, "Identifier"=w327:string, "Source"=w325:T16)  [unwired: 7 in]
            n117 = property class="VI"("Front Panel.Title"=w317) -> ()  [unwired: 2 in, 2 out]
            n118 = call "System Message.vi"("Sys. Msg. Source"=w325, "Payload"=w326, "Identifier"=w327) -> ()  [unwired: 8 in, 1 out]
            n119 = call "SM Request Transition.vi"("Req. Transition"=w329, "error in (no error)"=w331, "Transition"=SM_Transitions."Initialization finished") -> ("error out"=w330:errorcluster)  [unwired: 8 in]
            n120 = call "Module Name--constant.vi"() -> ("Module Name"=w332:string)  [unwired: 11 in]
            n121 = Format Into String(format string="Module %s started.", w332) -> (resulting string=w333:string)  [unwired: 2 in, 1 out]
            n122 = call <vilib>:"INFO.vi"("Message"=w333, "error in"=w330) -> ("error out"=w335:errorcluster)  [unwired: 9 in]
          }
          frame "Prepare" {
            # "#CodeNeeded\n1. Configure this Message Case for handling the \"Prepare\" message.\n2. Delete or edit this label when done."
            # "Prepare (the UI of the) module for display.\nIn this case  the FP can be updated BEFORE it is shown, if needed."
            n123 = property on="Request Transition" class="Enum (strict)"(error in=w339, "Value"=SM_Transitions."No Transition" ("Request Transition")) -> (error out=w338:errorcluster)  [unwired: 1 in, 1 out]
            n124 = Unbundle By Name(w343) -> ("Scenario"=w342:T5)
            n125 = control-ref of="This VI"() -> (w341:refnum<vi>)
            n126 = case shown="\"Stand-Alone\", Default" w342 {
              tunnel: w341 -> [w346 w349]
              tunnel: [w345 w348] -> w340
              tunnel: w338 -> [w344 w347]
              frame "Stand-Alone", Default {
                n127 = call "Open VI Panel.vi"("error in (no error)"=w344, "VI"=w346) -> ("error out"=w345:errorcluster)  [unwired: 9 in]
              }
              frame "Managed" {
                n128 = call "DQMH System Message - Ready for Display.vi"("Main VI Reference"=w349) -> ("Payload"=w351:variant, "Identifier"=w352:string, "Source"=w350:T16)  [unwired: 8 in]
                n129 = call "System Message.vi"("Sys. Msg. Source"=w350, "error in (no error)"=w347, "Payload"=w351, "Identifier"=w352) -> ("error out"=w348:errorcluster)  [unwired: 7 in]
              }
            }
          }
          frame "Request UI Display" {
            # "#CodeNeeded\n1. Decide if the module can be displayed or not.\n2. Adapt this case accordingly.\n3. Delete or edit this label when done."
            # "Requests the module to display its UI as specified in <b>Scenario</b>:\n\"managed\" => in the UI Manager's subpanel\n\"stand-alone\" => as a separate window"
            n130 = Variant To Data(error in=w366, type=T10 {"Scenario"=enum."Stand-Alone", "Wait Notifier"=refnum, "wait for reply"=FALSE} ("Request UI Display Argument"), Variant=w364) -> (data=w362:T10, error out=w355:errorcluster)
            n131 = Unbundle By Name(w362) -> ("Scenario"=w357:T5, "Wait Notifier"=w361:refnum<notifier>, "wait for reply"=w360:bool)
            n132 = Bundle By Name(cluster=w365, "Scenario"=w357) -> (w358:T4)
            n133 = call-poly <vilib>:"Delacor_lib_QMH_Enqueue Message (poly).vi"("error in"=w355, "Message"="Prepare", "Message Queue in"=w353) -> ("error out"=w354:errorcluster)  [unwired: 7 in, 1 out]
            n134 = Merge Errors(w354) -> (w359:errorcluster)
            n135 = case shown="True" w360 {
              tunnel: w361 -> [_ w370]
              frame False {
                # "Without reply."
              }
              frame True {
                # "With reply."
                n136 = Bundle By Name(cluster=T14 {"Accept?"=FALSE, "error"={"status"=FALSE, "code"=0, "source"=""}} ("Request UI Display (Reply Payload)"), "Accept?"=TRUE) -> (w369:T14)
                n137 = Send Notification(notification=w369, notifier=w370) -> ()  [unwired: 1 in, 2 out]
              }
            }
          }
          frame "--- Module Specific ---" {
            # "Separator -- The following cases handle messages specific to this Module."
          }
          frame "Update UI State" {
            w377 = SM_States."Initialising"  # State
            # "just for demo purposes"
            # "#CodeNeeded\nadd UI update code (show/hide or  enable/disable controls) as needed\ntell other modules, that this module will only stop depending on its state \ne.g. Set Application Closeable State To False"
            # "Updates the UI, i.e. sets control visibility, switches tab, etc., in accordance to the module's state"
            n138 = Variant To Data(error in=w379, type=w377, Variant=w376) -> (data=w373:T2, error out=w375:errorcluster)
            n139 = case shown="\"Error - Waiting For Action\", Default" w373 {
              tunnel: w375 -> [w382 w383 w386]
              tunnel: [w381 w383 w385] -> w374
              frame "Error - Waiting For Action", Default {
                n140 = call "Set Window Closeable State.vi"("error in (no error)"=w382, "Closeable?"=TRUE) -> ("error out"=w381:errorcluster)  [unwired: 9 in]
              }
              frame "Initialising" {
                # "re-initialise the polling control"
                n141 = local write "Polling Loop Signal"(FALSE ("Polling Loop Signal")) -> ()
              }
              frame "Waiting for External Trigger", "Polling for Signal Change" {
                # "In this stages the state machine \ndoesn't allow Exit transitions\n- inform the UI Manager"
                n142 = call "Set Window Closeable State.vi"("error in (no error)"=w386, "Closeable?"=FALSE) -> ("error out"=w385:errorcluster)  [unwired: 9 in]
              }
            }
            n143 = call "DEMO Updated UI State.vi"("State"=w373) -> ()  [unwired: 10 in, 1 out]
          }
          frame "---Example Functions for Show-Casing the SM---" {
            # "Duplicate this frame when creating new messages.  Change this comment in the duplicated frame to describe this message."
            n144 = Merge Errors(w390) -> (w389:errorcluster)
          }
          frame "DEMO Inject Transition" {
            # "Triggers a transition via the public API. \n\nThis request serves the purpose of testing/show-casing the state machine. By design, transitions should not be triggered from outside the DQMH module (i.e. via the public API)"
            n145 = Variant To Data(error in=w400, type=T11 {"Transition"=enum."No Transition", "Data"=variant} ("DEMO Inject Transition Argument"), Variant=w398) -> (data=w396:T11, error out=w395:errorcluster)
            n146 = Unbundle By Name(w396) -> ("Transition"=w393:T1, "Data"=w392:variant)
            n147 = case "Which transition was sent?" shown="Default" w393 {
              selector: w393 -> [_ w404]
              tunnel: w395 -> [w401 w406]
              tunnel: [w401 w405] -> w394
              tunnel: w392 -> [_ w403]
              tunnel: w391 -> [_ w402]
              frame "No Transition" {
                # "ignore the \"no transition\""
              }
              frame Default {
                # "forward any real transition"
                n148 = call "SM Request Transition.vi"("Req. Transition"=w402, "error in (no error)"=w406, "Data"=w403, "Transition"=w404) -> ("error out"=w405:errorcluster)  [unwired: 7 in]
              }
            }
          }
          frame "DEMO Exception Transition" {
            # "#HSE #ExceptionTransition"
            # "Example of how to manually call the \"Exception\" transition, which accepts an error cluster as its \"Data\" input"
            n149 = call "SM Request Transition.vi"("Req. Transition"=w409, "error in (no error)"=w408, "Data"=errorcluster {"status"=TRUE, "code"=654321, "source"="some error code"} ("error out"), "Transition"=SM_Transitions."Exception") -> ("error out"=w411:errorcluster)  [unwired: 7 in]
          }
          frame "--- Exit and Error Handling---" {
            # "Separator - The following cases handle errors and exit messages."
          }
          frame "Error" {
            # "Error - Check the error message data and respond accordingly. This message is sent by the \"Error Handler\" VIs at the end of each loop in this application."
            n150 = property class="Module Admin"(reference=w419) -> ("Accessors:External Launch"=w418:bool)  [unwired: 1 in, 2 out]
            n151 = Variant To Data(error in=w427, type=errorcluster {"status"=FALSE, "code"=0, "source"=""} ("error constant"), Variant=w421) -> (data=w416:errorcluster, error out=w425:errorcluster)
            n152 = call "Error Reported.vi"("Error"=w416) -> ()  [unwired: 10 in, 1 out]
            n153 = call <vilib>:"ERROR.vi"("Message"="DQMH Error Case", "error in"=w416) -> ("error out"=w415:errorcluster)  [unwired: 9 in]
            n154 = case shown="False" w418 {
              tunnel: [w432 _] -> w424
              tunnel: w420 -> [w430 _]
              tunnel: w415 -> [w431 _]
              frame False {
                # "If the module is running standalone, then pop up an error dialog and call the \"Exit\" message."
                n155 = call <vilib>:"Simple Error Handler.vi"("error in (no error)"=w431) -> ()  [unwired: 4 in, 5 out]
                n156 = call-poly <vilib>:"Delacor_lib_QMH_Enqueue Message (poly).vi"("Priority Message? (F)"=TRUE, "Message"="Exit", "Message Queue in"=w430) -> ("error out"=w432:errorcluster)  [unwired: 7 in, 1 out]
              }
              frame True {
                # "If the module was launched externally, calling the Error Reported broadcast VI is the only action performed by the \"Error\" message. The module's caller can then process the error appropriately."
              }
            }
            n157 = Merge Errors(w425, w424) -> (w423:errorcluster)
            n158 = local write "error out"(w423) -> ()
          }
          frame "Exit" {
            w434 = FALSE  # No confirmation (user cannot cancel)
            w447 = TRUE  # Stop the MHL Loop
            w441 = 91  # 91: not all Exit messages will have an argument
            # "Tell the whole application to shut down.\nSeeing as this module was started by the\nframework, stopping it will in turn stop\neverything."
            # "If the state machine loop initiated the\nexit action then tell the EHL it should\nstop, too."
            # "Release the message queue reference"
            # "Exit - Exit the application."
            n159 = Variant To Data(error in=w450, type=T6 {"Origin"="", "Exit via Stop Module Req?"=FALSE, "Wait for Module to stop?"=FALSE} ("Stop Argument"), Variant=w446) -> (data=w444:T6, error out=w440:errorcluster)
            n160 = call <vilib>:"Clear Errors.vi"("error in (no error)"=w440, "specific error code to clear (0: all)"=w441) -> ("error out"=w439:errorcluster)  [unwired: 4 in, 1 out]
            n161 = call-dynamic "Delacor_lib_QMH_Release Message Queue.vi"("error in"=w439, "Message Queue"=w442) -> ("error out"=w438:errorcluster)  [unwired: 9 in]
            n162 = control-ref of="This VI"() -> (w435:refnum<vi>)
            n163 = call "Exit EHL.vi"() -> ("error out"=w436:errorcluster)  [unwired: 11 in]
            n164 = call "Shutdown Application.vi"("User Confirm?"=w434) -> ("error out"=w433:errorcluster)  [unwired: 10 in]
            n165 = call "Handle Exit.vi"("Stop Argument"=w444, "Admin in"=w443, "VI reference"=w435) -> ("error out"=w437:errorcluster)  [unwired: 7 in, 1 out]
            n166 = Merge Errors(w436, w433, w438, w437) -> (w449:errorcluster)
            n167 = call "Error Reported.vi"("Error"=w449) -> ()  [unwired: 10 in, 1 out]
          }
          frame Default {
            # "'Default' case only runs if there is a message that isn't defined in any of the other cases.  Output a programming error."
            n168 = call "Module Name--constant.vi"() -> ("Module Name"=w451:string)  [unwired: 11 in]
            n169 = xnode "Error Ring"("parameter 0"=w452, "parameter 1"=w451) -> ("error out"=w456:errorcluster)
            n170 = Merge Errors(w454, w456) -> (w455:errorcluster)
          }
        }
        n171 = call-dynamic "Delacor_lib_QMH_Error Handler - Message Handling Loop.vi"("error in"=w293, "Message Queue in"=w283) -> ("dup error in"=w290:errorcluster)  [unwired: 8 in, 1 out]
      }
    }
    frame Error {
      # "Synchronize Caller Events.vi will inform Start Module.vi that the module has launched and will let the code calling Start Module.vi register for broadcasts and would permit the caller receive the broadcast that an error occurred at launch time."
      n172 = call-dynamic "Delacor_lib_QMH_Release Message Queue.vi"("error in"=w468, "Message Queue"=w466) -> ("error out"=w467:errorcluster)  [unwired: 9 in]
      n173 = call "Synchronize Caller Events.vi"("Singleton Module Admin in"=w469) -> ("error out"=w474:errorcluster)  [unwired: 9 in, 1 out]
      n174 = call "Module Name--constant.vi"() -> ("Module Name"=w472:string)  [unwired: 11 in]
      n175 = Format Into String(format string="An error occurred during initialization. %s is no longer running.", w472) -> (resulting string=w470:string)  [unwired: 2 in, 1 out]
      n176 = Merge Errors(w467, w474) -> (w475:errorcluster)
      n177 = call "Error Reported.vi"("Additional Information"=w470, "Error"=w475) -> ()  [unwired: 9 in, 1 out]
    }
  }
  n178 = Merge Errors(w26, w28) -> (w7:errorcluster)
  n179 = call "SM Destroy Event.vi"("error in (no error)"=w7, "Req. Transition Event"=w5) -> ("error out"=w6:errorcluster)  [unwired: 9 in]
  n180 = call "Close Module.vi"("error in (no error)"=w6, "Module Admin in"=w23) -> ("error out"=w4:errorcluster, "External Launch"=w2:bool, "Module Admin out"=w18:refnum<class "Delacor_lib_QMH_Module Admin.lvclass">)  [unwired: 7 in]
  n181 = Unregister For Events(event registration refnum=w1, error in=w4) -> (error out=w3:errorcluster)
  n182 = Unregister For Events(event registration refnum=w22, error in=w3) -> (error out=w15:errorcluster)
  n183 = case "External Launch?" shown="True" w2 {
    tunnel: w15 -> [_ w476]
    frame False {
    }
    frame True {
      n184 = case shown="No Error" w476 {
        frame No Error {
          n185 = invoke class="VI" method="FP.Close"() -> ()  [unwired: 3 in, 3 out]
        }
        frame Error {
          n186 = invoke class="VI" method="FP.Open"("Activate"=TRUE ("Activate?")) -> ()  [unwired: 4 in, 5 out]
        }
      }
    }
  }
  n187 = local write "Module Admin"(w18) -> ()
  n188 = call "Module Name--constant.vi"() -> ("Module Name"=w14:string)  [unwired: 11 in]
  n189 = Format Into String(format string="Module %s stopped.", w14) -> (resulting string=w17:string)  [unwired: 2 in, 1 out]
  n190 = call <vilib>:"INFO.vi"("Message"=w17, "error in"=w15) -> ("error out"=→"error out":errorcluster)  [unwired: 9 in]
